vi "Logging_PrepareLogfile.vi"(9 "Column Names":string[](array[string]), 10 "FilePostfix":string, 11 "Logging Directory":string) -> (0 "error out":errorcluster, 2 "Filename":string, 3 "Byte Stream File out":refnum<file>)   [LabVIEW 2014]
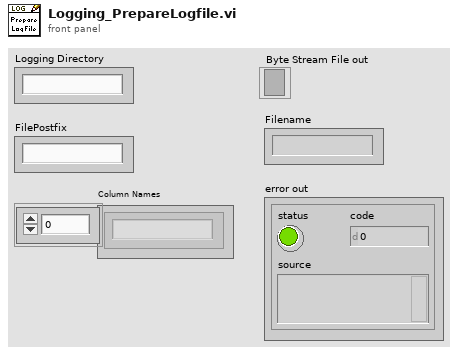
[diagram p1: front panel]
types:
  T1 = enum16{"open", "replace", "create", "open or create", "replace or create", "replace or create with confirmation"}
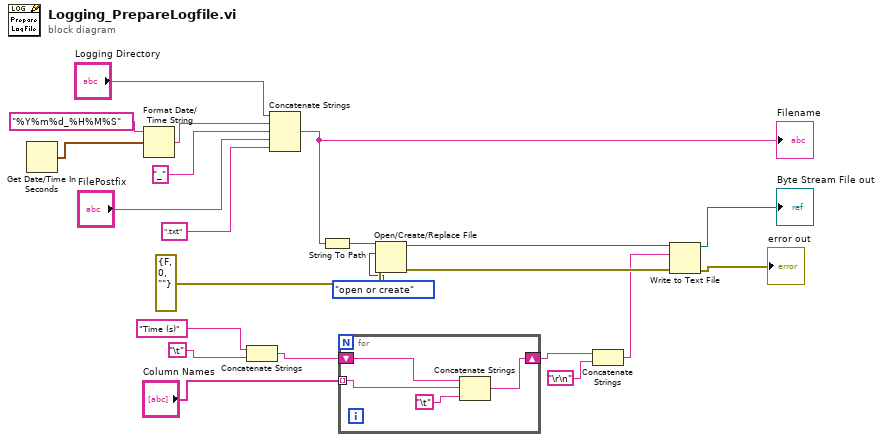
[diagram p0: block diagram]
diagram:
  n1 = Get Date/Time In Seconds() -> (seconds since 1Jan1904=w3:timestamp)
  n2 = Format Date/Time String(time format string (%c)="%Y%m%d_%H%M%S", seconds (now)=w3) -> (date/time string=w5:string)  [unwired: 1 out]
  n3 = Concatenate Strings("Time (s)", "\t") -> (w12:string)
  n4 = Concatenate Strings("Logging Directory", w5, "_" ("string"), "FilePostfix", ".txt" ("string")) -> (w6:string)
  "Filename" <- w6
  n5 = String To Path(string=w6) -> (path=w1:path)
  n6 = for {
    tunnel: "Column Names" -> [w23] mode=indexing
    shift-right: [w24] -> w11
    shift-left: w12 -> [w25]
    n7 = Concatenate Strings(w25, w23, "\t") -> (w24:string)
  }
  n8 = Open/Create/Replace File(file path (use dialog)=w1, error in=errorcluster {"status"=FALSE, "code"=0, "source"=""}, operation (0:open)=T1."open or create" ("opération (0 : open)")) -> (refnum out=w16:refnum<file>, error out=w21:errorcluster)  [unwired: 3 in, 1 out]
  n9 = Concatenate Strings(w11, "\r\n") -> (w9:string)
  n10 = Write to Text File(file (use dialog)=w16, text=w9, error in=w21) -> (refnum out=→"Byte Stream File out":refnum<file>, error out=→"error out":errorcluster)  [unwired: 1 in, 1 out]
